vi "NI-XNET Frame&Log - Get Frame Size.vi"(5 "raw frames":u8[](array[numeric]) format="%02x", 7 "index":i32) -> (6 "next index":i32=-1, 8 "size":i32, 10 "partial?":bool)   [LabVIEW 2014]
doc: "Get the size (in bytes) of the frame located at index in the raw frame data.\n\nIf the frame is not complete, then partial? is returned true. \n\nNext index is used for the next frame. If the current frame or next frame is incomplete, next index is -1."
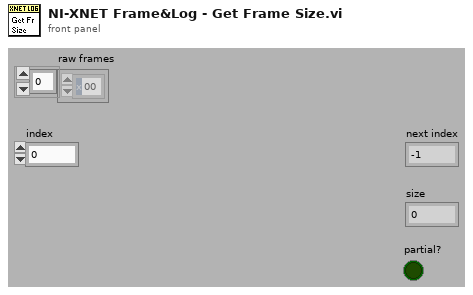
[diagram p1: front panel]
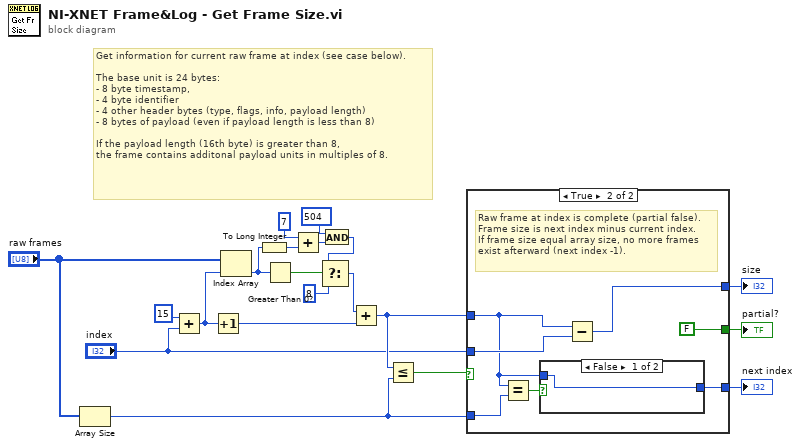
[diagram p0: block diagram]
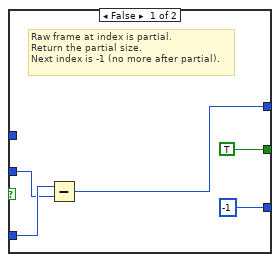
[diagram p2: hidden frame]
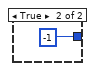
[diagram p3: hidden frame]
diagram:
  # "Get information for current raw frame at index (see case below).\n\nThe base unit is 24 bytes: \n- 8 byte timestamp,\n- 4 byte identifier\n- 4 other header bytes (type, flags, info, payload length)\n- 8 bytes of payload (even if payload length is less than 8)\n\nIf the payload length (16th byte) is greater than 8, \nthe frame contains additonal payload units in multiples of 8."
  n1 = Array Size(array="raw frames") -> (size(s)=w4:i32)
  n2 = Add(x=15 ("y"), y="index") -> (x+y=w14:i32)
  n3 = Increment(x=w14) -> (x+1=w12:i32)
  n4 = Index Array(array="raw frames", index=w14) -> (element=w11:u8)
  n5 = To Long Integer(number=w11) -> (32bit integer=w10:i32)
  n6 = Greater Than 0?(x=w11) -> (x > 0?=w20:bool)
  n7 = Add(x=7 ("y"), y=w10) -> (x+y=w17:i32)
  n8 = And(x=504 ("y"), y=w17) -> (x .and. y?=w15:i32)
  n9 = Select(t=w15, s=w20, f=8 ("y")) -> (s? t:f=w13:i32)
  n10 = Add(x=w13, y=w12) -> (x+y=w3:i32)
  n11 = Less Or Equal?(x=w3, y=w4) -> (x <= y?=w7:bool)
  n12 = case shown="True" w7 {
    tunnel: w3 -> [_ w26]
    tunnel: [-1 w31] -> w6
    tunnel: [TRUE ("partial?") FALSE ("partial?")] -> w5
    tunnel: w4 -> [w23 w32]
    tunnel: "index" -> [w22 w28]
    tunnel: [w24 w27] -> w1
    frame False {
      # "Raw frame at index is partial.\nReturn the partial size.\nNext index is -1 (no more after partial)."
      n13 = Subtract(x=w23, y=w22) -> (x-y=w24:i32)
    }
    frame True {
      # "Raw frame at index is complete (partial false).\nFrame size is next index minus current index.\nIf frame size equal array size, no more frames\nexist afterward (next index -1)."
      n14 = Equal?(x=w26, y=w32) -> (x = y?=w30:bool)
      n15 = case shown="False" w30 {
        tunnel: [w33 -1 ("next index")] -> w31
        tunnel: w26 -> [w33 _]
        frame False {
        }
        frame True {
        }
      }
      n16 = Subtract(x=w26, y=w28) -> (x-y=w27:i32)
    }
  }
  "next index" <- w6
  "partial?" <- w5
  "size" <- w1
